vi "Periodic Tasks.vi"(8 "error in":errorcluster) -> ()   [LabVIEW 2017]
doc: "This VI runs in parallel to other tasks. It can contain as many user-defined periodic loops as you need. These can carry out PID or other sorts of timed response."
uses:
  <vilib>/Rock Robotics/WPI/ThirdParty/Phoenix-LabVIEW/Motor Controller/Controls/CTRE_Phoenix_MotorControl_FeedbackDevice.ctl
  <vilib>/Rock Robotics/WPI/ThirdParty/Phoenix-LabVIEW/Motor Controller/Controls/CTRE_Phoenix_MotorControl_StatusFrameEnhanced.ctl
  <vilib>/Rock Robotics/WPI/ThirdParty/Phoenix-LabVIEW/Motor Controller/Controls/CTRE_Phoenix_MotorControl_ControlMode.ctl
  <vilib>/Rock Robotics/WPI/ThirdParty/Phoenix-LabVIEW/Motor Controller/Controls/CTRE_Phoenix_MotorControl_TrajectoryPointTimeDur.ctl
  <vilib>/Rock Robotics/WPI/Utilities/WPI_GetSetVariantRefNum.vi
  <vilib>/Utility/file.llb/Read Delimited Spreadsheet (DBL).vi
panel:
  out "Btm Mot Prof Count":i32
  out "Sensor Out Of Phase":bool
  out "Loop Time":u32
  out "Points in the CSV":i32
  out "Mot Prof Active Position":dbl
  out "Mot Prof Active Velocity":dbl
  out "Top Mot Prof Count":i32
  out "Mot Prof Active Is Valid":bool
  out "Mot Prof Active Is Last":bool
  out "Mot Prof  Has Under Run":bool
  out "Mot Prof  Is Under Run":bool
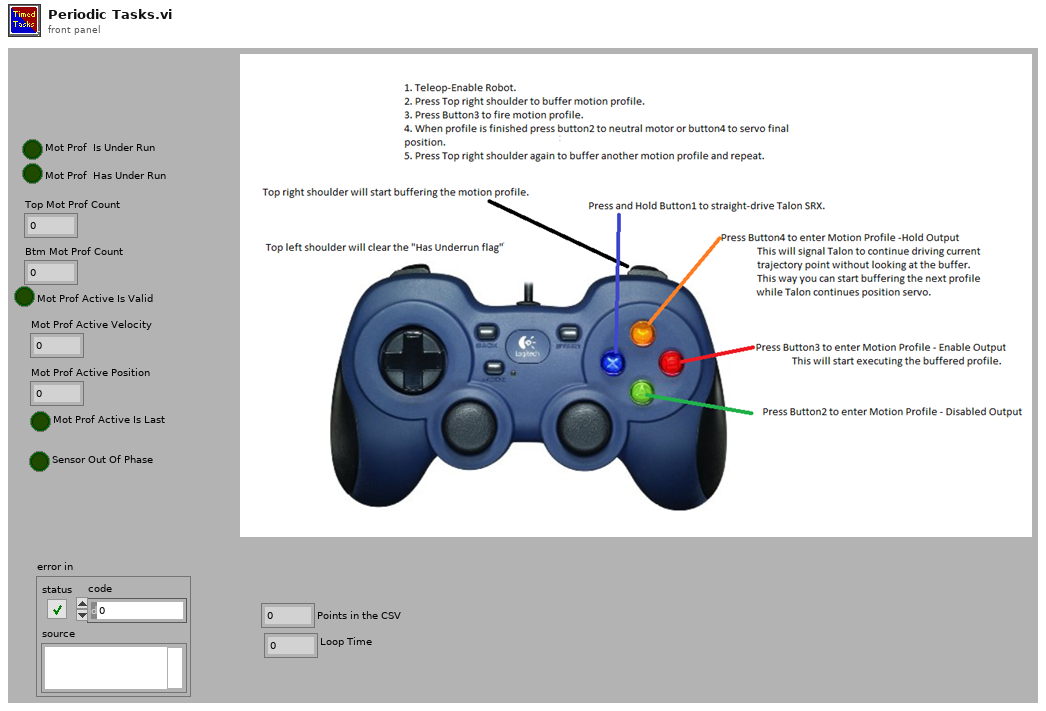
[diagram p1: front panel]
types:
  T1 = typedef "CTRE_Phoenix_MotorControl_StatusFrameEnhanced.ctl" = u16
  T2 = typedef "CTRE_Phoenix_MotorControl_FeedbackDevice.ctl" = i8
  T3 = typedef "WPI_MotorControlDeviceRef.ctl" = cluster{"DeviceStatus":errorcluster, "Type":T4, "PWM":cluster{"PWM Channel":T5, "DeadBand":T6}, "CAN":cluster{"Device Number":u8, "SetOutput VI Ref":variant, "GetOutput VI Ref":variant, "Enable VI Ref":variant, "Disable VI Ref":variant, "Data":variant}, "Invert":bool, "DIO PWM":cluster{"PWM \"Enable\" Channel":T5, "DIOChannel":T7, "PWM Rate":dbl}}
  T4 = typedef "WPI_MotorControlType.ctl" = enum16{"PWM", "CAN", "DIO PWM"}
  T5 = typedef "FPGA_DIOPWMChannel.ctl" = enum8{"PWM 0", "PWM 1", "PWM 2", "PWM 3", "PWM 4", "PWM 5", "PWM 6", "PWM 7", "PWM 8", "PWM 9", "PWM MXP 0", "PWM MXP 1", "PWM MXP 2", "PWM MXP 3", "PWM MXP 4", "PWM MXP 5", "PWM MXP 6", "PWM MXP 7", "PWM MXP 8", "PWM MXP 9", "Invalid"}
  T6 = typedef "WPI_PWMDeadband.ctl" = cluster{"Name":string, "maxPositivePwm":i32, "minPositivePwm":i32, "centerPwm":i32, "maxNegativePwm":i32, "minNegativePwm":i32, "angularRange":u16}
  T7 = typedef "FPGA_DIOChannel.ctl" = enum8{"DIO 0", "DIO 1", "DIO 2", "DIO 3", "DIO 4", "DIO 5", "DIO 6", "DIO 7", "DIO 8", "DIO 9", "DIO MXP 0", "DIO MXP 1", "DIO MXP 2", "DIO MXP 3", "DIO MXP 4", "DIO MXP 5", "DIO MXP 6", "DIO MXP 7", "DIO MXP 8", "DIO MXP 9", "DIO MXP 10", "DIO MXP 11", "DIO MXP 12", "DIO MXP 13", "DIO MXP 14", "DIO MXP 15", "SPI Port CS1", "SPI Port CS2", "SPI Port CS3", "SPI Port MISO", "SPI Port MOSI", "Invalid"}
  T8 = typedef "WPI_JoystickDevRef.ctl" = cluster{"Device":T9}
  T9 = typedef "WPI_JoystickDeviceEnum.ctl" = enum16{"USB 0", "USB 1", "USB 2", "USB 3", "USB 4", "USB 5"}
  T10 = typedef "CTRE_Phoenix_MotorControl_ControlMode.ctl" = u16
  T11 = cluster{"Under Voltage":bool, "Forward Limit Switch":bool, "Reverse Limit Switch":bool, "Forward Soft Limit":bool, "Reverse Soft Limit":bool, "Hardware Failure":bool, "Reset During Enable":bool, "Sensor Overflow":bool, "Sensor Out of Phase":bool, "Hardware ESD Reset":bool, "Remote Loss of Signal":bool}
  T12 = cluster{"Top Buffer Remaining":i32, "Top Buffer Count":i32, "Bottom Buffer Count":i32, "Has Underrun?":bool, "Is Underrun?":bool, "Active Point Valid?":bool, "Is Last?":bool, "Profile Slot Select 0":i32, "Output Enable":i32, "Time Duration (ms)":i32, "Profile Slot Select 1":i32}
  T13 = typedef "CTRE_Phoenix_MotorControl_TrajectoryPointTimeDur.ctl" = i32
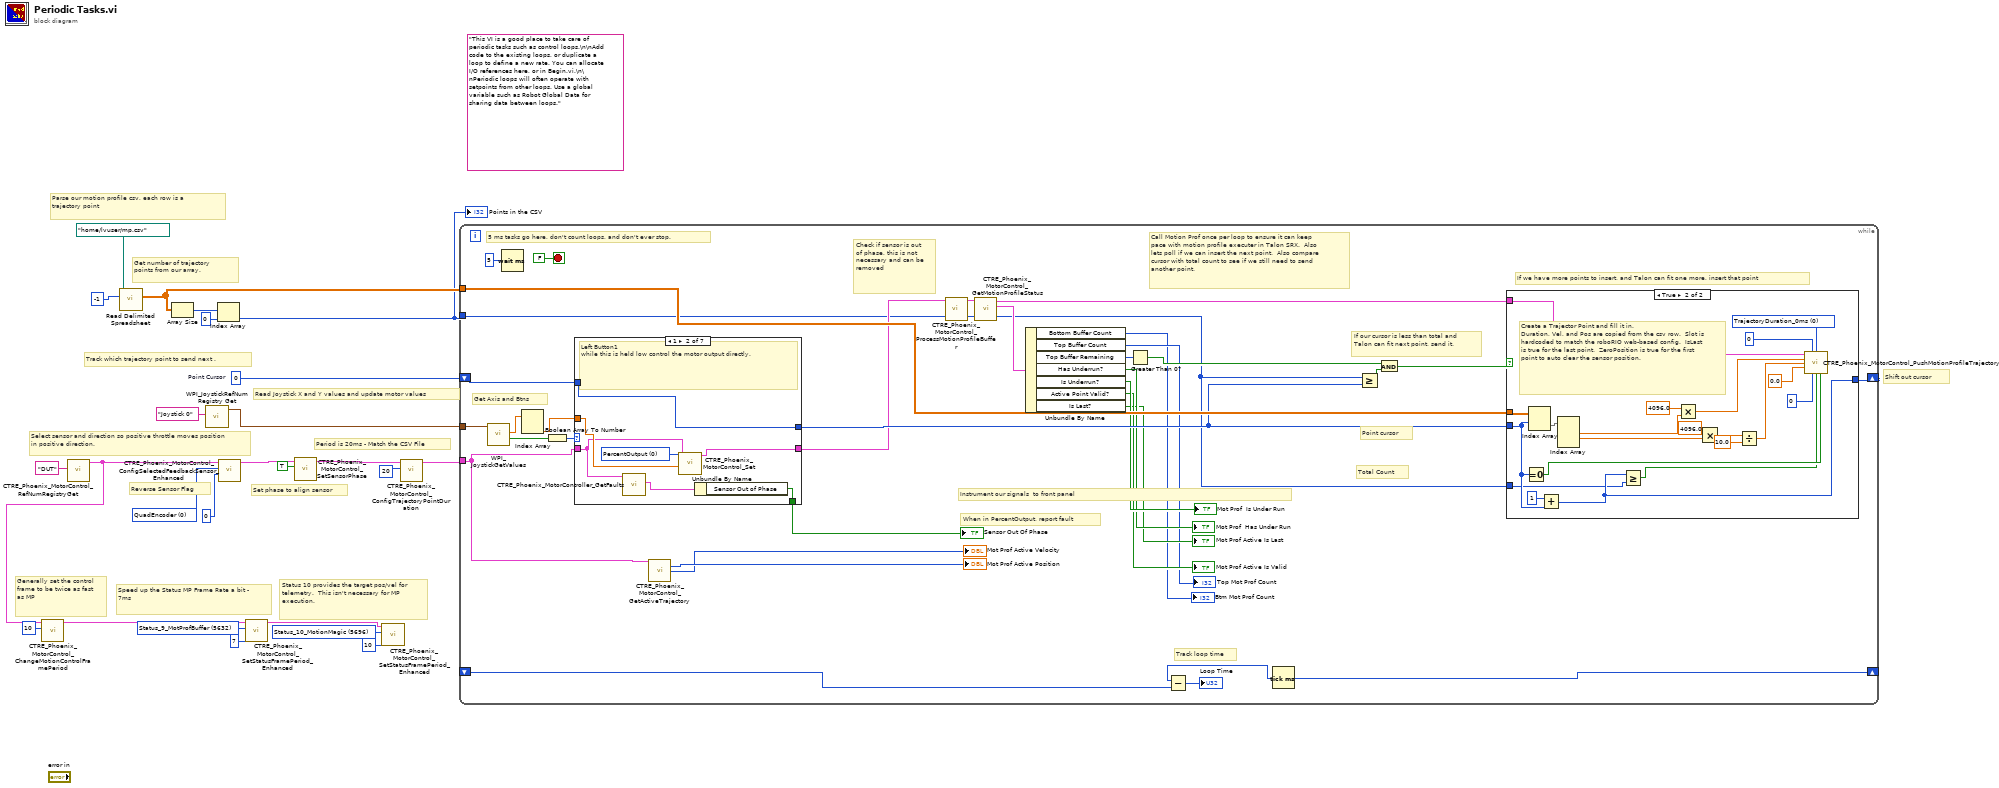
[diagram p0: block diagram]
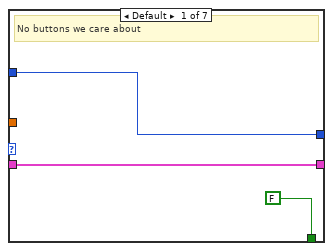
[diagram p2: hidden frame]
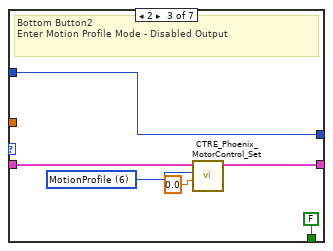
[diagram p3: hidden frame]
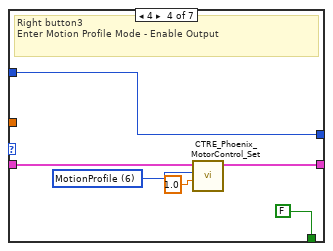
[diagram p4: hidden frame]
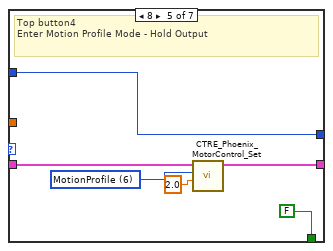
[diagram p5: hidden frame]
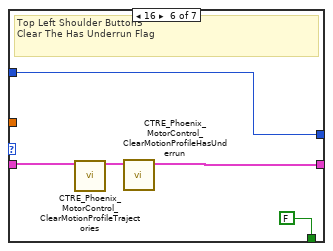
[diagram p6: hidden frame]
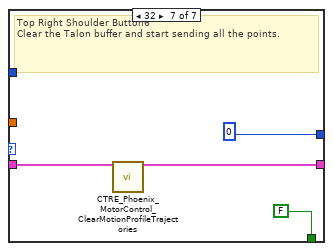
[diagram p7: hidden frame]
diagram:
  w9 = T1 5696 items=["Status_1_General"=5120, "Status_2_Feedback0"=5184, "Status_3_Quadrature"=5248, "Status_4_AinTempVbat"=5312, "Status_6_Misc"=5440, "Status_7_CommStatus"=5504, "Status_8_PulseWidth"=5568, "Status_9_MotProfBuffer"=5632, "Status_10_MotionMagic"=5696, "Status_11_UartGadgeteer"=5760, "Status_12_Feedback1"=5824, "Status_13_Base_PIDF0"=5888, "Status_14_Turn_PIDF1"=5952, "Status_15_FirmwareApiStatus"=6016] ("Status Frame")
  w13 = T1 5632 items=["Status_1_General"=5120, "Status_2_Feedback0"=5184, "Status_3_Quadrature"=5248, "Status_4_AinTempVbat"=5312, "Status_6_Misc"=5440, "Status_7_CommStatus"=5504, "Status_8_PulseWidth"=5568, "Status_9_MotProfBuffer"=5632, "Status_10_MotionMagic"=5696, "Status_11_UartGadgeteer"=5760, "Status_12_Feedback1"=5824, "Status_13_Base_PIDF0"=5888, "Status_14_Turn_PIDF1"=5952, "Status_15_FirmwareApiStatus"=6016] ("Status Frame")
  w15 = T2 0 items=["None"=-1, "QuadEncoder"=0, "Analog"=2, "Tachometer"=4, "Pulse Width Encoded Position"=8, "Sensor Sum (S0 + S1)"=9, "Sensor Difference (D0 - D1)"=10, "Remote Source 0"=11, "Remote Source 1"=12, "Software Emulated"=15] ("Feedback Device")
  w20 = 0  # Point Cursor
  (unwired) "This VI is a good place to take care of periodic tasks such as control loops.\n\nAdd code to the existing loops, or duplicate a loop to define a new rate. You can allocate I/O references here, or in Begin.vi.\n\nPeriodic loops will often operate with setpoints from other loops. Use a global variable such as Robot Global Data for sharing data between loops."
  # "Set phase to align sensor"
  # "Generally set the control frame to be twice as fast as MP"
  # "Status 10 provides the target pos/vel for telemetry.  This isn't necessary for MP execution."
  # "Period is 20ms - Match the CSV File"
  # "Shift out cursor"
  # "Read Joystick X and Y values and update motor values"
  # "Reverse Sensor Flag"
  # "Select sensor and direction so positive throttle moves position in positive direction."
  # "Get number of trajectory points from our array."
  # "Track which trajectory point to send next ."
  # "Speed up the Status MP Frame Rate a bit - 7ms"
  # "Parse our motion profile csv, each row is a trajectory point"
  n1 = call <vilib>:"CTRE_Phoenix_MotorControl_RefNumRegistryGet.vi"("refnum name"="DUT") -> ("PhoenixMotorControlDevRef"=w4:T3)  [unwired: 9 in, 1 out]
  n2 = call <vilib>:"CTRE_Phoenix_MotorControl_ChangeMotionControlFramePeriod.vi"("periodMs"=10, "PhoenixMotorControlDevRef"=w4) -> ("PhoenixMotorControlDevRef"=w3:T3)  [unwired: 8 in, 1 out]
  n3 = call-poly <vilib>:"Read Delimited Spreadsheet.vi"("file path (dialog if empty)"=path "/home/lvuser/mp.csv" ("file path (use dialog)"), "number of rows (all:-1)"=-1) -> ("all rows"=w17:dbl[][])  [unwired: 8 in, 5 out]
  n4 = Array Size(array=w17) -> (size(s)=w18:i32[])
  n5 = call <vilib>:"WPI_JoystickRefNum Registry Get.vi"("refnum name"="Joystick 0") -> ("JoystickDevRef"=w23:T8)  [unwired: 1 in, 9 out]
  n6 = Index Array(array=w18, index=0) -> (element=w16:i32)
  "Points in the CSV" <- w16
  n7 = call <vilib>:"CTRE_Phoenix_MotorControl_ConfigSelectedFeedbackSensor_Enhanced.vi"("pidLoopIdx"=0, "Feedback Device"=w15, "PhoenixMotorControlDevRef"=w4) -> ("PhoenixMotorControlDevRef"=w11:T3)  [unwired: 7 in, 1 out]
  n8 = call <vilib>:"CTRE_Phoenix_MotorControl_SetStatusFramePeriod_Enhanced.vi"("periodMs"=7, "Status Frame"=w13, "PhoenixMotorControlDevRef"=w3) -> ("PhoenixMotorControlDevRef"=w7:T3)  [unwired: 7 in, 1 out]
  n9 = call <vilib>:"CTRE_Phoenix_MotorControl_SetSensorPhase.vi"("PhaseSensor"=TRUE, "PhoenixMotorControlDevRef"=w11) -> ("PhoenixMotorControlDevRef"=w5:T3)  [unwired: 8 in, 1 out]
  n10 = call <vilib>:"CTRE_Phoenix_MotorControl_SetStatusFramePeriod_Enhanced.vi"("periodMs"=10, "Status Frame"=w9, "PhoenixMotorControlDevRef"=w7) -> ()  [unwired: 7 in, 2 out]
  n11 = call <vilib>:"CTRE_Phoenix_MotorControl_ConfigTrajectoryPointDuration.vi"("durationMs"=20 ("periodMs"), "PhoenixMotorControlDevRef"=w5) -> ("PhoenixMotorControlDevRef"=w6:T3)  [unwired: 8 in, 1 out]
  n12 = while {
    tunnel: w23 -> [w56]
    tunnel: w17 -> [w55]
    shift-right: [w54] -> _
    shift-left: w20 -> [w53]
    tunnel: w16 -> [w26]
    tunnel: w6 -> [w30]
    shift-right: [w33] -> _
    shift-left: _ -> [w32]
    stop <- FALSE stop-if-true
    # "Track loop time"
    # "When in PercentOutput, report fault"
    # "Check if sensor is out of phase, this is not necessary and can be removed"
    # "Call Motion Prof once per loop to ensure it can keep pace with motion profile executer in Talon SRX.  Also lets poll if we can insert the next point.  Also compare cursor with total count to see if we still need to send another point."
    # "Instrument our signals  to front panel"
    # "Get Axis and Btns"
    # "Point cursor"
    # "Total Count"
    # "If our cursor is less than total and Talon can fit next point, send it."
    # "If we have more points to insert, and Talon can fit one more, insert that point"
    # "5 ms tasks go here, don't count loops, and don't ever stop."
    n13 = call <vilib>:"WPI_JoystickGetValues.vi"("JoystickDevRef"=w56) -> ("Buttons"=w46:bool[], "Axes"=w47:dbl[])  [unwired: 6 in, 3 out]
    n14 = Wait (ms)(milliseconds to wait=u32 5) -> ()  [unwired: 1 out]
    n15 = Index Array(array=w47) -> (element #2=w44:dbl)  [unwired: 2 in, 1 out]
    n16 = Boolean Array To Number(Boolean array=w46) -> (number=w45:u32)
    n17 = case shown="1" w45 {
      tunnel: w30 -> [w61 w65 w72 w78 w86 w89 w93]
      tunnel: [w61 w63 w71 w77 w83 w90 w94] -> w28
      tunnel: w44 -> [_ w68 _ _ _ _ _]
      tunnel: [w60 w67 w70 w76 w82 w91 0 ("Capacity")] -> w51
      tunnel: w53 -> [w60 w67 w70 w76 w82 w91 _]
      tunnel: [FALSE ("Sensor Out of Phase") w62 FALSE ("Sensor Out of Phase") FALSE ("Sensor Out of Phase") FALSE ("Sensor Out of Phase") FALSE ("Sensor Out of Phase") FALSE ("Sensor Out of Phase")] -> w27
      frame Default {
        # "No buttons we care about"
      }
      frame 1 {
        w66 = T10 0 items=["PercentOutput"=0, "Position"=1, "Velocity"=2, "Current"=3, "Follower"=5, "MotionProfile"=6, "MotionMagic"=7, "MotionMagicArc"=8, "MotionProfileArc"=10, "Disabled"=15] ("Control Mode")
        # "Left Button1\nwhile this is held low control the motor output directly."
        n18 = call <vilib>:"CTRE_Phoenix_MotorController_GetFaults.vi"("PhoenixMotorControlDevRef"=w65) -> ("Faults"=w64:T11)  [unwired: 8 in, 2 out]
        n19 = call <vilib>:"CTRE_Phoenix_MotorControl_Set.vi"("Output"=w68, "Control Mode"=w66, "PhoenixMotorControlDevRef"=w65) -> ("PhoenixMotorControlDevRef"=w63:T3)  [unwired: 7 in, 1 out]
        n20 = Unbundle By Name(w64) -> ("Sensor Out of Phase"=w62:bool)
      }
      frame 2 {
        w74 = T10 6 items=["PercentOutput"=0, "Position"=1, "Velocity"=2, "Current"=3, "Follower"=5, "MotionProfile"=6, "MotionMagic"=7, "MotionMagicArc"=8, "MotionProfileArc"=10, "Disabled"=15] ("Control Mode")
        # "Bottom Button2\nEnter Motion Profile Mode - Disabled Output"
        n21 = call <vilib>:"CTRE_Phoenix_MotorControl_Set.vi"("Output"=0.0, "Control Mode"=w74, "PhoenixMotorControlDevRef"=w72) -> ("PhoenixMotorControlDevRef"=w71:T3)  [unwired: 7 in, 1 out]
      }
      frame 4 {
        w80 = T10 6 items=["PercentOutput"=0, "Position"=1, "Velocity"=2, "Current"=3, "Follower"=5, "MotionProfile"=6, "MotionMagic"=7, "MotionMagicArc"=8, "MotionProfileArc"=10, "Disabled"=15] ("Control Mode")
        # "Right button3\nEnter Motion Profile Mode - Enable Output"
        n22 = call <vilib>:"CTRE_Phoenix_MotorControl_Set.vi"("Output"=1.0, "Control Mode"=w80, "PhoenixMotorControlDevRef"=w78) -> ("PhoenixMotorControlDevRef"=w77:T3)  [unwired: 7 in, 1 out]
      }
      frame 8 {
        w85 = T10 6 items=["PercentOutput"=0, "Position"=1, "Velocity"=2, "Current"=3, "Follower"=5, "MotionProfile"=6, "MotionMagic"=7, "MotionMagicArc"=8, "MotionProfileArc"=10, "Disabled"=15] ("Control Mode")
        # "Top button4\nEnter Motion Profile Mode - Hold Output"
        n23 = call <vilib>:"CTRE_Phoenix_MotorControl_Set.vi"("Output"=2.0, "Control Mode"=w85, "PhoenixMotorControlDevRef"=w86) -> ("PhoenixMotorControlDevRef"=w83:T3)  [unwired: 7 in, 1 out]
      }
      frame 16 {
        # "Top Left Shoulder Button5\nClear The Has Underrun Flag"
        n24 = call <vilib>:"CTRE_Phoenix_MotorControl_ClearMotionProfileTrajectories.vi"("PhoenixMotorControlDevRef"=w89) -> ("PhoenixMotorControlDevRef"=w88:T3)  [unwired: 13 in, 1 out]
        n25 = call <vilib>:"CTRE_Phoenix_MotorControl_ClearMotionProfileHasUnderrun.vi"("PhoenixMotorControlDevRef"=w88) -> ("PhoenixMotorControlDevRef"=w90:T3)  [unwired: 9 in, 1 out]
      }
      frame 32 {
        # "Top Right Shoulder Button6\nClear the Talon buffer and start sending all the points."
        n26 = call <vilib>:"CTRE_Phoenix_MotorControl_ClearMotionProfileTrajectories.vi"("PhoenixMotorControlDevRef"=w93) -> ("PhoenixMotorControlDevRef"=w94:T3)  [unwired: 13 in, 1 out]
      }
    }
    "Sensor Out Of Phase" <- w27
    n27 = call <vilib>:"CTRE_Phoenix_MotorControl_GetActiveTrajectory.vi"("PhoenixMotorControlDevRef"=w30) -> ("Position (Sensor Units)"=→"Mot Prof Active Position":i32, "Velocity (Sensor Units per 100 ms)"=→"Mot Prof Active Velocity":i32)  [unwired: 10 in, 3 out]
    n28 = call <vilib>:"CTRE_Phoenix_MotorControl_ProcessMotionProfileBuffer.vi"("PhoenixMotorControlDevRef"=w28) -> ("PhoenixMotorControlDevRef"=w41:T3)  [unwired: 13 in, 1 out]
    n29 = call <vilib>:"CTRE_Phoenix_MotorControl_GetMotionProfileStatus.vi"("PhoenixMotorControlDevRef"=w41) -> ("Motion Profile Status"=w43:T12, "PhoenixMotorControlDevRef"=w49:T3)  [unwired: 8 in, 1 out]
    n30 = Unbundle By Name(w43) -> ("Bottom Buffer Count"=→"Btm Mot Prof Count":i32, "Top Buffer Count"=→"Top Mot Prof Count":i32, "Top Buffer Remaining"=w42:i32, "Has Underrun?"=→"Mot Prof  Has Under Run":bool, "Is Underrun?"=→"Mot Prof  Is Under Run":bool, "Active Point Valid?"=→"Mot Prof Active Is Valid":bool, "Is Last?"=→"Mot Prof Active Is Last":bool)
    n31 = Greater Than 0?(x=w42) -> (x > 0?=w48:bool)
    n32 = Tick Count (ms)() -> (millisecond timer value=w33:u32)
    n33 = Subtract(x=w33, y=w32) -> (x-y=→"Loop Time":u32)
    n34 = Greater Or Equal?(x=w26, y=w51) -> (x >= y?=w50:bool)
    n35 = And(x=w48, y=w50) -> (x .and. y?=w52:bool)
    n36 = case shown="True" w52 {
      tunnel: w55 -> [_ w117]
      tunnel: [w96 w113] -> w54
      tunnel: w51 -> [w96 w114]
      tunnel: w26 -> [_ w112]
      tunnel: w49 -> [_ w111]
      frame False {
      }
      frame True {
        w98 = T13 0 items=["TrajectoryDuration_0ms"=0, "TrajectoryDuration_5ms"=5, "TrajectoryDuration_10ms"=10, "TrajectoryDuration_20ms"=20, "TrajectoryDuration_30ms"=30, "TrajectoryDuration_40ms"=40, "TrajectoryDuration_50ms"=50, "TrajectoryDuration_100ms"=100] ("durationMs")
        # "Create a Trajector Point and fill it in.\nDuration, Vel, and Pos are copied from the csv row.  Slot is hardcoded to match the roboRIO web-based config.  IsLast is true for the last point.  ZeroPosition is true for the first point to auto clear the sensor position."
        n37 = Equal To 0?(x=w114) -> (x = 0?=w109:bool)
        n38 = Index Array(array=w117, index (row)=w114) -> (element=w115:dbl[])  [unwired: 1 in]
        n39 = Add(x=u32 1, y=w114) -> (x+y=w113:u32)
        n40 = Index Array(array=w115) -> (element #1=w105:dbl, element #2=w102:dbl)  [unwired: 3 in, 1 out]
        n41 = Greater Or Equal?(x=w113, y=w112) -> (x >= y?=w108:bool)
        n42 = Multiply(x=4096.0, y=w105) -> (x*y=w104:dbl)
        n43 = Multiply(x=4096.0, y=w102) -> (x*y=w100:dbl)
        n44 = Divide(x=w100, y=10.0) -> (x/y=w99:dbl)
        n45 = call <vilib>:"CTRE_Phoenix_MotorControl_PushMotionProfileTrajectory.vi"("PhoenixMotorControlDevRef"=w111, "profileSlotSelect1"=0, "durationMs"=w98, "position"=w104, "velocity"=w99, "auxiliaryPos"=0.0 ("headingDeg"), "profileSlotSelect0"=0, "isLastPoint?"=w108, "Zero Position?"=w109) -> ()  [unwired: 5 in, 2 out]
      }
    }
  }
